vi "DrawBlobRect.vi"(1 "BlobLineDataArray":T2(array[cluster]), 2 "Dest In":T1, 3 "Src In":T1) -> (0 "Image Out":T1)   [LabVIEW 2011]
uses:
  <vilib>/vision/Image Controls.llb/IMAQ Image.ctl
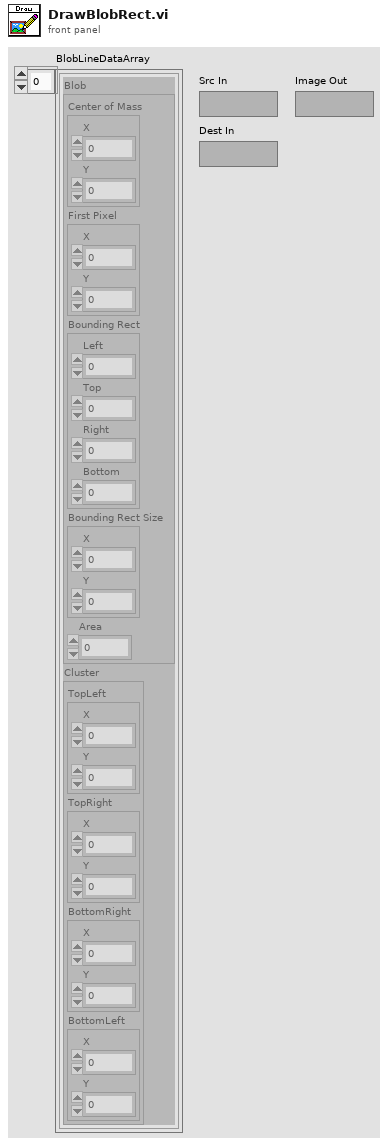
[diagram p1: front panel]
types:
  T1 = typedef "IMAQ Image.ctl" = refnum<image>
  T2 = cluster{"Blob":cluster{"Center of Mass":cluster{"X":dbl, "Y":dbl}, "First Pixel":cluster{"X":dbl, "Y":dbl}, "Bounding Rect":cluster{"Left":dbl, "Top":dbl, "Right":dbl, "Bottom":dbl}, "Bounding Rect Size":cluster{"X":dbl, "Y":dbl}, "Area":dbl}, "Cluster":cluster{"TopLeft":cluster{"X":dbl, "Y":dbl}, "TopRight":cluster{"X":dbl, "Y":dbl}, "BottomRight":cluster{"X":dbl, "Y":dbl}, "BottomLeft":cluster{"X":dbl, "Y":dbl}}}[]
  T3 = typedef "Image Type" = u32
  T4 = cluster{"Center of Mass":cluster{"X":dbl, "Y":dbl}, "First Pixel":cluster{"X":dbl, "Y":dbl}, "Bounding Rect":cluster{"Left":dbl, "Top":dbl, "Right":dbl, "Bottom":dbl}, "Bounding Rect Size":cluster{"X":dbl, "Y":dbl}, "Area":dbl}
  T5 = cluster{"TopLeft":cluster{"X":dbl, "Y":dbl}, "TopRight":cluster{"X":dbl, "Y":dbl}, "BottomRight":cluster{"X":dbl, "Y":dbl}, "BottomLeft":cluster{"X":dbl, "Y":dbl}}
  T6 = cluster{"Left":dbl, "Top":dbl, "Right":dbl, "Bottom":dbl}
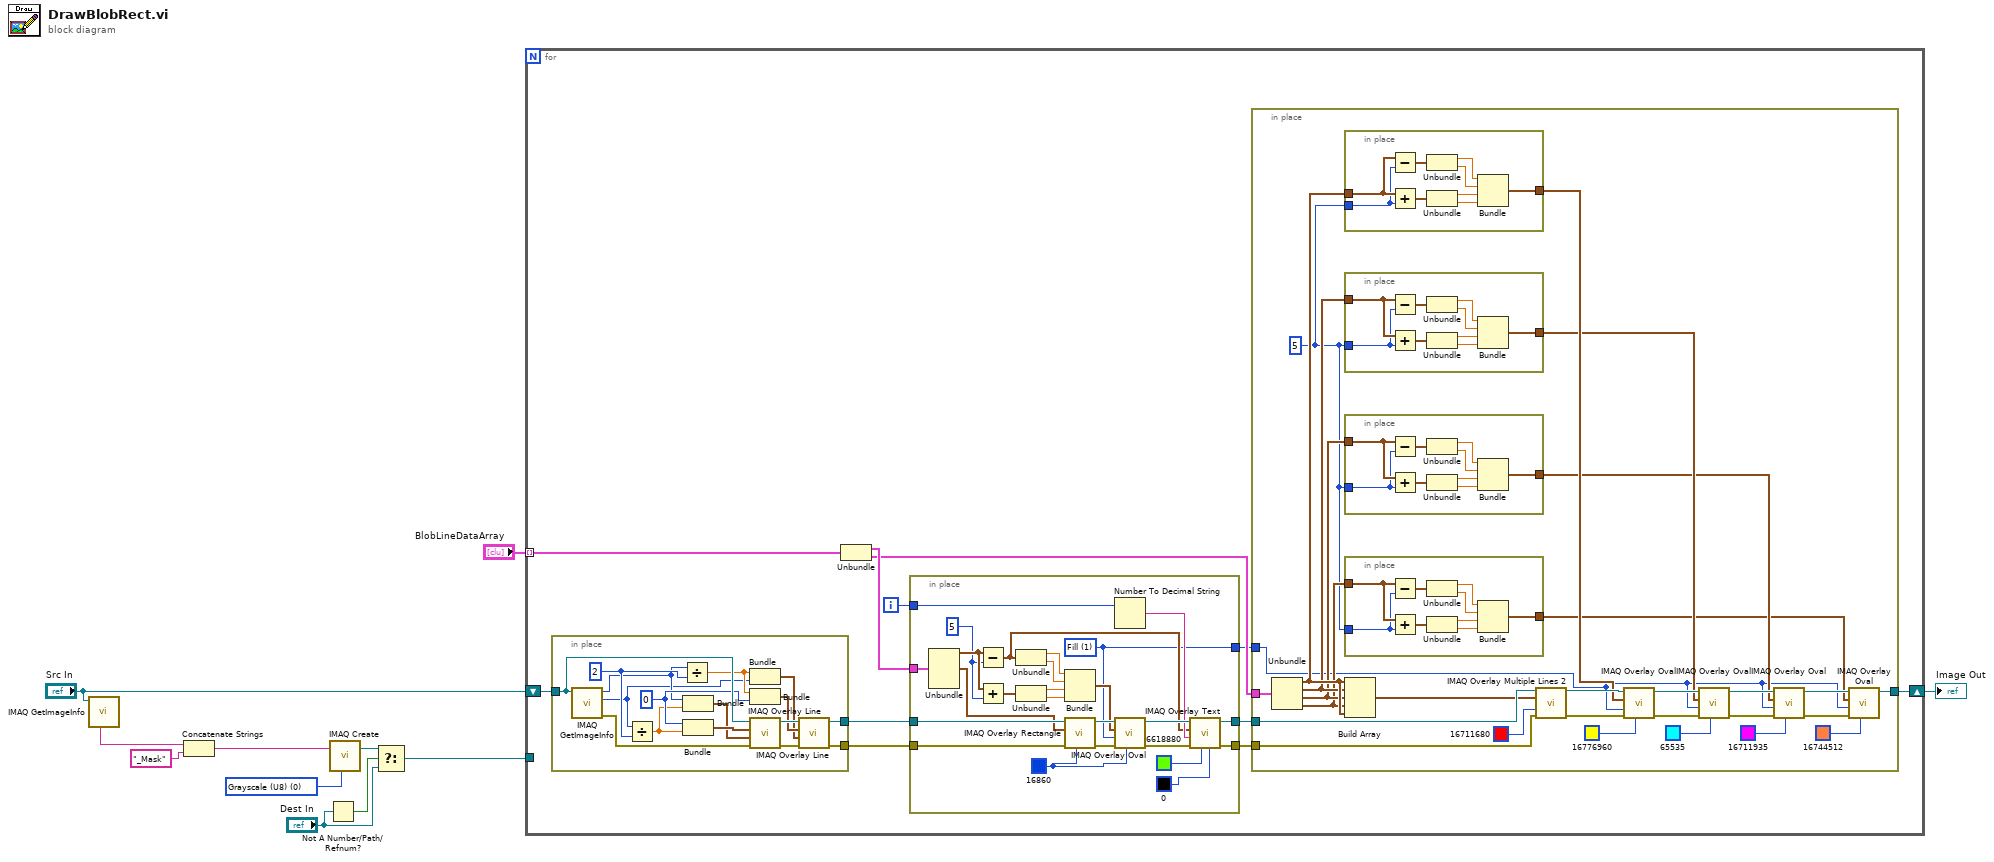
[diagram p0: block diagram]
diagram:
  w1 = T3 0 items=["Grayscale (U8)", "Grayscale (I16)", "Grayscale (SGL)", "Complex (CSG)", "RGB (U32)", "HSL (U32)", "RGB (U64)", "Grayscale (U16)"] ("Image Type")
  n1 = call "IMAQ GetImageInfo"("Image"="Src In") -> ("Image Name"=w5:string)  [unwired: 3 in, 7 out]
  n2 = Concatenate Strings(w5, "_Mask" ("string")) -> (w3:string)
  n3 = Not A Number/Path/Refnum?(number/path/refnum="Dest In") -> (NaN/Path/Refnum?=w9:bool)
  n4 = call "IMAQ Create"("Image Name"=w3, "Image Type"=w1) -> ("New Image"=w6:T1)  [unwired: 3 in, 1 out]
  n5 = Select(t=w6, s=w9, f="Dest In") -> (s? t:f=w7:T1)
  n6 = for {
    tunnel: "BlobLineDataArray" -> [w22] mode=indexing
    shift-right: [w16] -> w10
    shift-left: "Src In" -> [w14]
    tunnel: w7 -> [_]
    i -> [w20]
    n7 = in-place {
      in-place-border: w14 -> [w35]
      in-place-border: [w24] -> w13
      in-place-border: [w23] -> w12
      w33 = 2 ("y")
      w34 = 0
      n8 = call "IMAQ GetImageInfo"("Image"=w35) -> ("error out"=w36:errorcluster, "Y Resolution"=w29:i32, "X Resolution"=w31:i32)  [unwired: 3 in, 5 out]
      n9 = Divide(x=w29, y=w33) -> (x/y=w32:dbl)
      n10 = Divide(x=w31, y=w33) -> (x/y=w30:dbl)
      n11 = Bundle("X Resolution"=w31, w32) -> (w27:cluster{"X Resolution":i32, dbl})  [unwired: 1 in]
      n12 = Bundle(w34, w32) -> (w28:cluster{i32, dbl})  [unwired: 1 in]
      n13 = Bundle(w30, "Y Resolution"=w29) -> (w25:cluster{dbl, "Y Resolution":i32})  [unwired: 1 in]
      n14 = Bundle(w30, w34) -> (w26:cluster{dbl, i32})  [unwired: 1 in]
      n15 = call "IMAQ Overlay Line"("error in (no error)"=w36, "End Point"=w27, "Start Point"=w28, "Image"=w35) -> ("error out"=w38:errorcluster, "Image Out"=w37:T1)  [unwired: 6 in]
      n16 = call "IMAQ Overlay Line"("error in (no error)"=w38, "End Point"=w25, "Start Point"=w26, "Image"=w37) -> ("error out"=w23:errorcluster, "Image Out"=w24:T1)  [unwired: 6 in]
    }
    n17 = Unbundle(w22) -> ("Blob"=w21:T4, "Cluster"=w17:T5)
    n18 = in-place {
      in-place-border: w21 -> [w127]
      in-place-border: w13 -> [w126]
      in-place-border: w20 -> [w111]
      in-place-border: [w106] -> w19
      in-place-border: [w105] -> w18
      in-place-border: [w104] -> w15
      in-place-border: w12 -> [w103]
      w114 = u32 16860 ("Color")
      w104 = u32 1 items=["Frame", "Fill"] ("Drawing Mode (Frame)")
      w121 = 5
      n19 = Unbundle(w127) -> ("Center of Mass"=w122:cluster{"X":dbl, "Y":dbl}, "Bounding Rect"=w125:T6)  [unwired: 3 out]
      n20 = Subtract(x=w122, y=w121) -> (x-y=w109:cluster{"X":dbl, "Y":dbl})
      n21 = Add(x=w122, y=w121) -> (x+y=w120:cluster{"X":dbl, "Y":dbl})
      n22 = Unbundle(w109) -> ("X"=w119:dbl, "Y"=w118:dbl)
      n23 = Unbundle(w120) -> ("X"=w117:dbl, "Y"=w116:dbl)
      n24 = Bundle("X"=w119, "Y"=w118, "X"=w117, "Y"=w116) -> (w115:cluster{"X":dbl, "Y":dbl, "X":dbl, "Y":dbl})  [unwired: 1 in]
      n25 = call "IMAQ Overlay Rectangle"("Color"=w114, "error in (no error)"=w103, "Rectangle"=w125, "Image"=w126) -> ("error out"=w124:errorcluster, "Image Out"=w123:T1)  [unwired: 6 in]
      n26 = Number To Decimal String(number=w111) -> (decimal integer string=w110:string)  [unwired: 1 in]
      n27 = call "IMAQ Overlay Oval"("Color"=w114, "error in (no error)"=w124, "Drawing Mode (Frame)"=w104, "Bounding Rectangle"=w115, "Image"=w123) -> ("error out"=w113:errorcluster, "Image Out"=w112:T1)  [unwired: 5 in]
      n28 = call "IMAQ Overlay Text"("BG Color (Transparent)"=u32 0, "Text Color (black)"=u32 6618880, "error in (no error)"=w113, "String"=w110, "Origin"=w109, "Image"=w112) -> ("error out"=w105:errorcluster, "Image Out"=w106:T1)  [unwired: 4 in]
    }
    n29 = in-place {
      in-place-border: w19 -> [w66]
      in-place-border: w18 -> [w65]
      in-place-border: w17 -> [w64]
      in-place-border: [w53] -> w16
      in-place-border: w15 -> [w44]
      w58 = 5
      n30 = Unbundle(w64) -> ("TopLeft"=w62:cluster{"X":dbl, "Y":dbl}, "TopRight"=w61:cluster{"X":dbl, "Y":dbl}, "BottomRight"=w60:cluster{"X":dbl, "Y":dbl}, "BottomLeft"=w59:cluster{"X":dbl, "Y":dbl})
      n31 = in-place {
        in-place-border: w62 -> [w96]
        in-place-border: [w95] -> w48
        in-place-border: w58 -> [w94]
        n32 = Subtract(x=w96, y=w94) -> (x-y=w102:cluster{"X":dbl, "Y":dbl})
        n33 = Add(x=w96, y=w94) -> (x+y=w97:cluster{"X":dbl, "Y":dbl})
        n34 = Unbundle(w102) -> ("X"=w98:dbl, "Y"=w99:dbl)
        n35 = Unbundle(w97) -> ("X"=w100:dbl, "Y"=w101:dbl)
        n36 = Bundle("X"=w98, "Y"=w99, "X"=w100, "Y"=w101) -> (w95:cluster{"X":dbl, "Y":dbl, "X":dbl, "Y":dbl})  [unwired: 1 in]
      }
      n37 = in-place {
        in-place-border: w61 -> [w87]
        in-place-border: [w86] -> w47
        in-place-border: w58 -> [w85]
        n38 = Subtract(x=w87, y=w85) -> (x-y=w93:cluster{"X":dbl, "Y":dbl})
        n39 = Add(x=w87, y=w85) -> (x+y=w88:cluster{"X":dbl, "Y":dbl})
        n40 = Unbundle(w93) -> ("X"=w89:dbl, "Y"=w90:dbl)
        n41 = Unbundle(w88) -> ("X"=w91:dbl, "Y"=w92:dbl)
        n42 = Bundle("X"=w89, "Y"=w90, "X"=w91, "Y"=w92) -> (w86:cluster{"X":dbl, "Y":dbl, "X":dbl, "Y":dbl})  [unwired: 1 in]
      }
      n43 = in-place {
        in-place-border: w60 -> [w78]
        in-place-border: [w77] -> w46
        in-place-border: w58 -> [w76]
        n44 = Subtract(x=w78, y=w76) -> (x-y=w84:cluster{"X":dbl, "Y":dbl})
        n45 = Add(x=w78, y=w76) -> (x+y=w79:cluster{"X":dbl, "Y":dbl})
        n46 = Unbundle(w84) -> ("X"=w80:dbl, "Y"=w81:dbl)
        n47 = Unbundle(w79) -> ("X"=w82:dbl, "Y"=w83:dbl)
        n48 = Bundle("X"=w80, "Y"=w81, "X"=w82, "Y"=w83) -> (w77:cluster{"X":dbl, "Y":dbl, "X":dbl, "Y":dbl})  [unwired: 1 in]
      }
      n49 = in-place {
        in-place-border: w59 -> [w69]
        in-place-border: [w68] -> w45
        in-place-border: w58 -> [w67]
        n50 = Subtract(x=w69, y=w67) -> (x-y=w75:cluster{"X":dbl, "Y":dbl})
        n51 = Add(x=w69, y=w67) -> (x+y=w70:cluster{"X":dbl, "Y":dbl})
        n52 = Unbundle(w75) -> ("X"=w71:dbl, "Y"=w72:dbl)
        n53 = Unbundle(w70) -> ("X"=w73:dbl, "Y"=w74:dbl)
        n54 = Bundle("X"=w71, "Y"=w72, "X"=w73, "Y"=w74) -> (w68:cluster{"X":dbl, "Y":dbl, "X":dbl, "Y":dbl})  [unwired: 1 in]
      }
      n55 = Build Array(w62, w61, w60, w59, w62) -> (w63:cluster{"X":dbl, "Y":dbl}[])
      n56 = call "IMAQ Overlay Multiple Lines 2"("Image"=w66, "Line End Points"=w63, "Color"=u32 16711680, "error in (no error)"=w65) -> ("Image Out"=w57:T1, "error out"=w49:errorcluster)  [unwired: 10 in]
      n57 = call "IMAQ Overlay Oval"("Color"=u32 16776960, "error in (no error)"=w49, "Drawing Mode (Frame)"=w44, "Bounding Rectangle"=w48, "Image"=w57) -> ("error out"=w52:errorcluster, "Image Out"=w56:T1)  [unwired: 5 in]
      n58 = call "IMAQ Overlay Oval"("Color"=u32 65535, "error in (no error)"=w52, "Drawing Mode (Frame)"=w44, "Bounding Rectangle"=w47, "Image"=w56) -> ("error out"=w51:errorcluster, "Image Out"=w55:T1)  [unwired: 5 in]
      n59 = call "IMAQ Overlay Oval"("Color"=u32 16711935, "error in (no error)"=w51, "Drawing Mode (Frame)"=w44, "Bounding Rectangle"=w46, "Image"=w55) -> ("error out"=w50:errorcluster, "Image Out"=w54:T1)  [unwired: 5 in]
      n60 = call "IMAQ Overlay Oval"("Color"=u32 16744512, "error in (no error)"=w50, "Drawing Mode (Frame)"=w44, "Bounding Rectangle"=w45, "Image"=w54) -> ("Image Out"=w53:T1)  [unwired: 5 in, 1 out]
    }
  }
  "Image Out" <- w10
